vi "Compare.vi"(1 "Banking Record Y":refnum<class "Banking Record.lvclass">, 2 "Banking Record X":refnum<class "Banking Record.lvclass">) -> (0 "Equal?":bool)   [LabVIEW 2018, in "Banking Record.lvclass"]
uses:
  Banking Record.lvclass
  Banking Record.lvclass/Banking Record.ctl
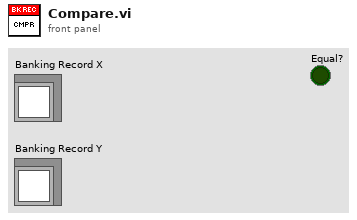
[diagram p1: front panel]
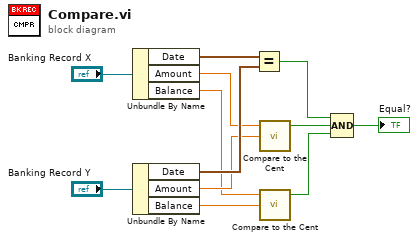
[diagram p0: block diagram]
diagram:
  n1 = Unbundle By Name("Banking Record X") -> ("Date"=w8:timestamp, "Amount"=w6:dbl, "Balance"=w3:dbl)
  n2 = Unbundle By Name("Banking Record Y") -> ("Date"=w7:timestamp, "Amount"=w5:dbl, "Balance"=w2:dbl)
  n3 = Equal?(x=w8, y=w7) -> (x = y?=w10:bool)
  n4 = call "Compare to the Cent.vi"("Dollar y"=w5, "Dollar x"=w6) -> ("x = y?"=w4:bool)  [unwired: 3 in]
  n5 = call "Compare to the Cent.vi"("Dollar y"=w2, "Dollar x"=w3) -> ("x = y?"=w1:bool)  [unwired: 3 in]
  n6 = Compound Arithmetic op=AND(w10, w4, w1) -> (→"Equal?":bool)
